vi "Perform Action.vi"(8 "Error In":errorcluster, 10 "Input":variant, 11 "reference in":refnum<class "Instrument.lvclass">) -> (0 "Error Out":errorcluster, 2 "Output":variant, 3 "reference out":refnum<class "Instrument.lvclass">)   [LabVIEW 2024, in "HAL.lvlib" / "Instrument.lvclass"]
uses:
  Instrument.lvclass
  Instrument.lvclass/Instrument.ctl
  Configurations/CFG Base/CFG Base.lvclass
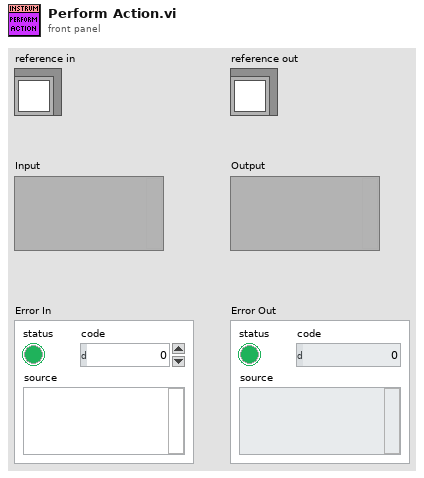
[diagram p1: front panel]
types:
  T1 = typedef "HAL.lvlib/Instrument.lvclass/ObjectAttributes.ctl" = cluster{"CFG Base":refnum<class "CFG Base.lvclass">, "Started Counter":i16}
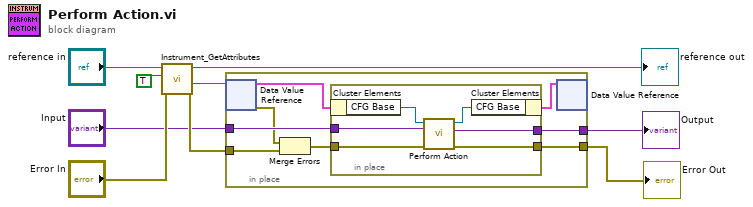
[diagram p0: block diagram]
diagram:
  n1 = call "Instrument_GetAttributes.vi"("Error In"="Error In", "OnlyGetDvrReference(False)"=TRUE, "reference in"="reference in") -> ("Error Out"=w5:errorcluster, "DataRef"=w1:refnum<data-value>, "reference out"=→"reference out":refnum<class "Instrument.lvclass">)  [unwired: 5 in, 1 out]
  n2 = in-place {
    in-place-border: w5 -> [w17]
    in-place-border: [w16] -> w4
    in-place-border: "Input" -> [w15]
    in-place-border: [w14] -> w2
    n3 = in-place-dvr #1(w1) -> (w13:T1, w11:errorcluster)
    n4 = Merge Errors(w11, w17) -> (w12:errorcluster)
    n5 = in-place {
      in-place-border: w12 -> [w23]
      in-place-border: [w22] -> w16
      in-place-border: w15 -> [w21]
      in-place-border: [w20] -> w14
      n6 = in-place-cluster #2(w13) -> ("CFG Base"=w19:refnum<class "CFG Base.lvclass">)
      n7 = call-dynamic "Perform Action.vi"("error in"=w23, "Input"=w21, "CFG Base in"=w19) -> ("error out"=w22:errorcluster, "Output"=w20:variant, "CFG Base out"=w18:refnum<class "CFG Base.lvclass">)  [unwired: 6 in]
      n8 = in-place-cluster #2("CFG Base"=w18) -> (w10:T1)
    }
    n9 = in-place-dvr #1(w10) -> ()  [unwired: 2 out]
  }
  "Error Out" <- w4
  "Output" <- w2
